vi "Read Path Section.vi"(7 "LC Type":T1, 8 "error in (no error)":errorcluster, 11 "FP-TC-Shared in":refnum<class "FP-TC-Shared.lvclass">) -> (0 "error out":errorcluster, 2 "Paths":string[](array[string]), 3 "FP-TC-Shared out":refnum<class "FP-TC-Shared.lvclass">)   [LabVIEW 2019, in "FP-TC-Shared.lvclass"]
uses:
  FP-TC-Shared.lvclass
  typedefs/LC Type--Enum.ctl
  FP-TC-Shared.lvclass/FP-TC-Shared.ctl
  <vilib>/Utility/config.llb/NI_LVConfig.lvlib
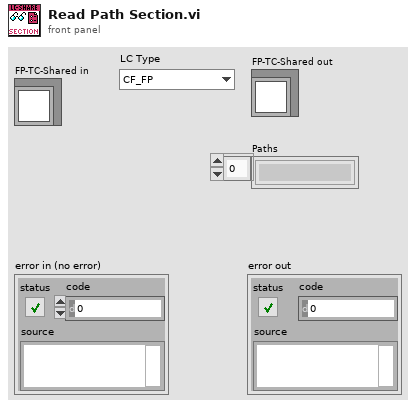
[diagram p1: front panel]
types:
  T1 = typedef "FP-TC-Shared.lvclass/LC Type--Enum.ctl" = enum16{"CF_FP", "CF_TC", "CF_TC_Z", "MNK_FP", "MNK_TC", "MNK_TC_Z"}
  T2 = typedef "NI_LVConfig.lvlib/Config Data RefNum.ctl" = refnum<k1>
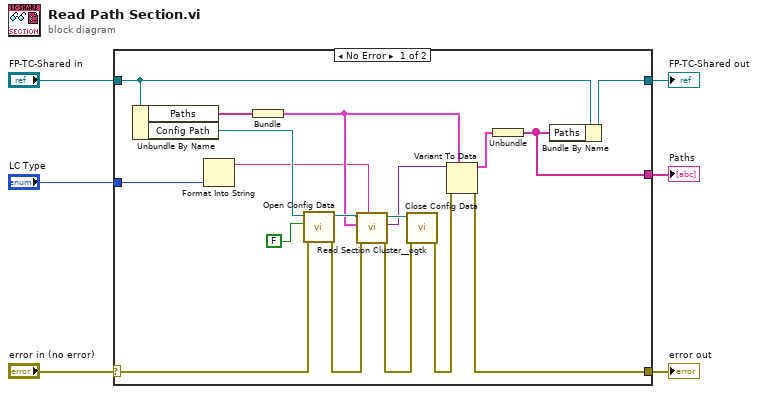
[diagram p0: block diagram]
diagram:
  n1 = case shown="No Error" "error in (no error)" {
    selector: "error in (no error)" -> [w24 w26]
    tunnel: "FP-TC-Shared in" -> [w16 w25]
    tunnel: [w15 w25] -> w4
    tunnel: [w13 w26] -> w3
    tunnel: [w10 _] -> w2
    tunnel: "LC Type" -> [w9 _]
    frame No Error {
      n2 = Unbundle By Name(w16) -> ("Paths"=w7:string[], "Config Path"=w23:path)
      n3 = Format Into String(w9) -> (resulting string=w8:string)  [unwired: 3 in, 1 out]
      n4 = Bundle("Paths"=w7) -> (w18:cluster{"Paths":string[]})  [unwired: 1 in]
      n5 = call <vilib>:"Open Config Data.vi"("error in (no error)"=w24, "create file if necessary (T)"=FALSE, "configuration file path"=w23) -> ("error out"=w19:errorcluster, "refnum"=w20:T2)  [unwired: 6 in, 1 out]
      n6 = call <userlib>:"Read Section Cluster__ogtk.vi"("section (optional)"=w8, "error in (no error)"=w19, "Section Formatted Cluster Type"=w18, "refnum"=w20) -> ("error out"=w21:errorcluster, "Section Formatted Cluster"=w17:variant, "dup refnum"=w22:T2)  [unwired: 3 in, 2 out]
      n7 = call <vilib>:"Close Config Data.vi"("error in (no error)"=w21, "refnum"=w22) -> ("error out"=w14:errorcluster)  [unwired: 8 in, 1 out]
      n8 = Variant To Data(error in=w14, type=w18, Variant=w17) -> (data=w11:cluster{"Paths":string[]}, error out=w13:errorcluster)
      n9 = Unbundle(w11) -> ("Paths"=w10:string[])
      n10 = Bundle By Name(cluster=w16, "Paths"=w10) -> (w15:refnum<class "FP-TC-Shared.lvclass">)
    }
    frame Error {
    }
  }
  "Paths" <- w2
  "error out" <- w3
  "FP-TC-Shared out" <- w4
